vi "Read Data from Buffer.vi"(8 "error in (no error)":errorcluster, 11 "Hardware in":refnum<class "Hardware.lvclass">) -> (0 "error out":errorcluster, 2 "Variant":variant, 3 "Hardware out":refnum<class "Hardware.lvclass">)   [LabVIEW 2026, in "Hardware.lvlib" / "Hardware.lvclass"]
uses:
  Hardware.lvclass
  Hardware.lvclass/Hardware.ctl
  <vilib>/Utility/error.llb/Error Cluster From Error Code.vi
  <vilib>/ErrorRing/Error Ring.xnode
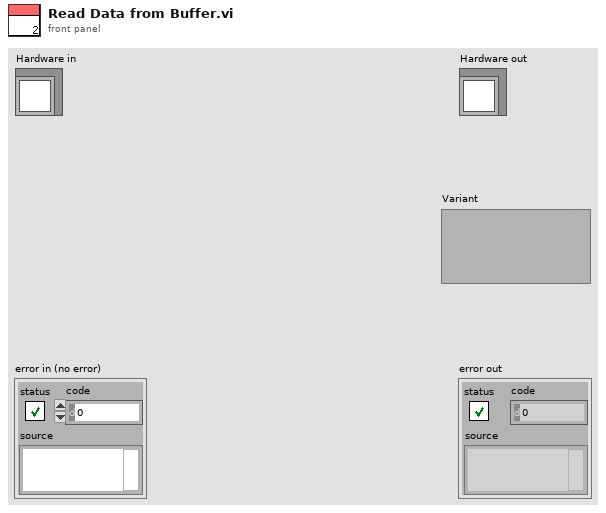
[diagram p1: front panel]
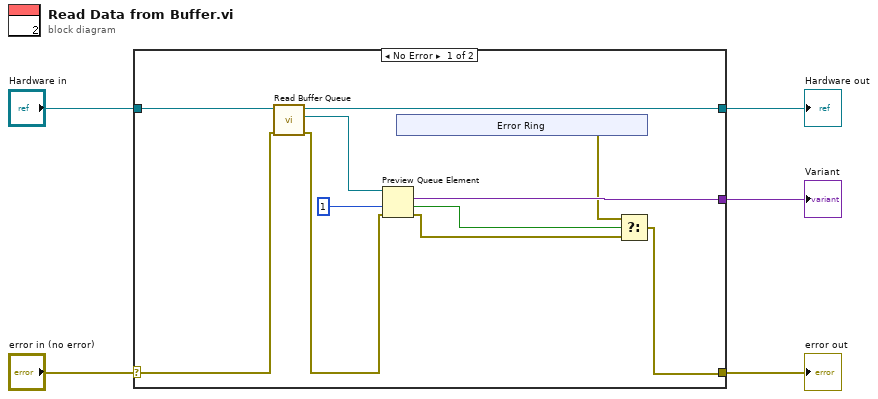
[diagram p0: block diagram]
diagram:
  n1 = case shown="No Error" "error in (no error)" {
    selector: "error in (no error)" -> [w13 w23]
    tunnel: [w6 w23] -> w4
    tunnel: [w14 w22] -> w2
    tunnel: "Hardware in" -> [w15 w22]
    tunnel: [w12 _] -> w1
    frame No Error {
      n2 = call "Read Buffer Queue.vi"("error in (no error)"=w13, "Hardware in"=w15) -> ("error out"=w11:errorcluster, "Buffer Queue"=w16:refnum<queue>, "Hardware out"=w14:refnum<class "Hardware.lvclass">)  [unwired: 7 in]
      n3 = Preview Queue Element(queue=w16, timeout in ms (-1)=1, error in (no error)=w11) -> (element=w12:variant, timed out?=w9:bool, error out=w8:errorcluster)  [unwired: 1 out]
      n4 = xnode "Error Ring"() -> ("error out"=w7:errorcluster)
      n5 = Select(t=w7, s=w9, f=w8) -> (s? t:f=w6:errorcluster)
    }
    frame Error {
    }
  }
  "error out" <- w4
  "Hardware out" <- w2
  "Variant" <- w1
